vi "uService GUI.vi"(8 "error in (no error)":errorcluster, 11 "uService Test in":refnum<class "test_us.lvclass">) -> (3 "uService Test out":refnum<class "test_us.lvclass">)   [LabVIEW 2026, in "test_us.lvlib" / "test_us.lvclass"]
uses:
  test_us.lvclass
  C:/LabVIEW Code/TALOS/talos/Father of all uServices/Father of all uServices/Father of all uServices.lvclass
  Ancestor/Ancestor/Ancestor.lvclass/Ancestor.ctl
  Support VIs/Substitute Error.vi
  Support VIs/Generate Error.vi
  FGV/Error Memory/Get Error Description.vi
  Support VIs/Get PC name.vi
  Ancestor/Ancestor/Read ID.vi
  Support VIs/Get Class Name.vi
  FGV/Error Memory/Error Memory Core.vi
  <vilib>/AdvancedString/Delimited String to 1D String Array.vi
  <vilib>/AdvancedString/Delimited String to 1D String Array (string).vi
  Support VIs/Circus Root Path.vi
  FGV/Error Memory/Error Crt Lvl checker.vi
  FGV/Error Memory/Error Memory Core.vi/40c8088d-b597-4017-91af-faa98e00292e.vi
  FGV/Error Memory/Error Memory Core.vi/d4a3ab98-063c-4e44-b43d-fbdcfe6c2be2.vi
  Father of all uServices/Father of all uServices/Father of all uServices.lvclass
  C:/LabVIEW Code/TALOS/builds/Actor Framework PPL/Actor Framework.lvlibp/1abvi3w/vi.lib/ActorFramework/Actor/Actor.lvclass
  builds/Actor Framework PPL/Actor Framework.lvlibp/1abvi3w/vi.lib/ActorFramework/Actor/Read Self Enqueuer.vi
  builds/Actor Framework PPL/Actor Framework.lvlibp/1abvi3w/vi.lib/ActorFramework/Stop Msg/Send Normal Stop.vi
  Support VIs/Global Memory.vi
  <vilib>/Utility/LVClass/Get LV Class Name.vi
  Support VIs/Is in Packed Library.vi
  Support VIs/TALOS Root path.vi
  Support VIs/Read CSV worksheet.vi
  Support VIs/Global Constants.vi
  <vilib>/Utility/error.llb/General Error Handler.vi
  Support VIs/Error Log.vi
  Ancestor/Ancestor/Ancestor.lvclass
  <vilib>/Comparison/Equal/Equal Functor/Equal Functor.lvclass
panel:
  in  "stop New uService":bool
  in  "Tab Control":T1(tab)
  in  "Send I exist":bool
  in  "Stop Pat":bool
  in  "Set Guardian Dead":bool
  in  "Snooze VI":bool
  in  "Switch uS View":bool
  out "Message Received":string
  in  "Message to myself":string
  in  "Send":bool
  in  "SEND to Guardian":bool
  in  "Delayed message":bool
  in  "Delay [s]":dbl
  out "Delay submit time":timestamp format="%<%x %.3X>T"
  out "Delay executed":timestamp format="%<%x %.3X>T"
  out "Test Infinite Message":u32
  in  "Start Infinite":bool
  in  "Check Infinite":bool
  in  "Stop Infinite":bool
  out "Infinite?":bool
  in  "send error":bool
  in  "error":errorcluster
  in  "Error code to filter":i32
  in  "Repetitions":i32
  in  "Time (s)":dbl
  in  "Filter error":bool
  in  "Update Run Number":bool
  in  "Run Number":u32
  in  "Send to DAQ":bool
  in  "Add point":bool
  out "LED":bool
  out "Waveform Chart":waveform(dbl)(graph)
  in  "Reset Graph":bool
  out "Counter":dbl
  in  "Set N":bool
  in  "N":i32
  in  "Read N":bool
  out "N out":i32
  out "Safe Mode":bool
  out "uService ID":string
  # "I'm the test uService!"
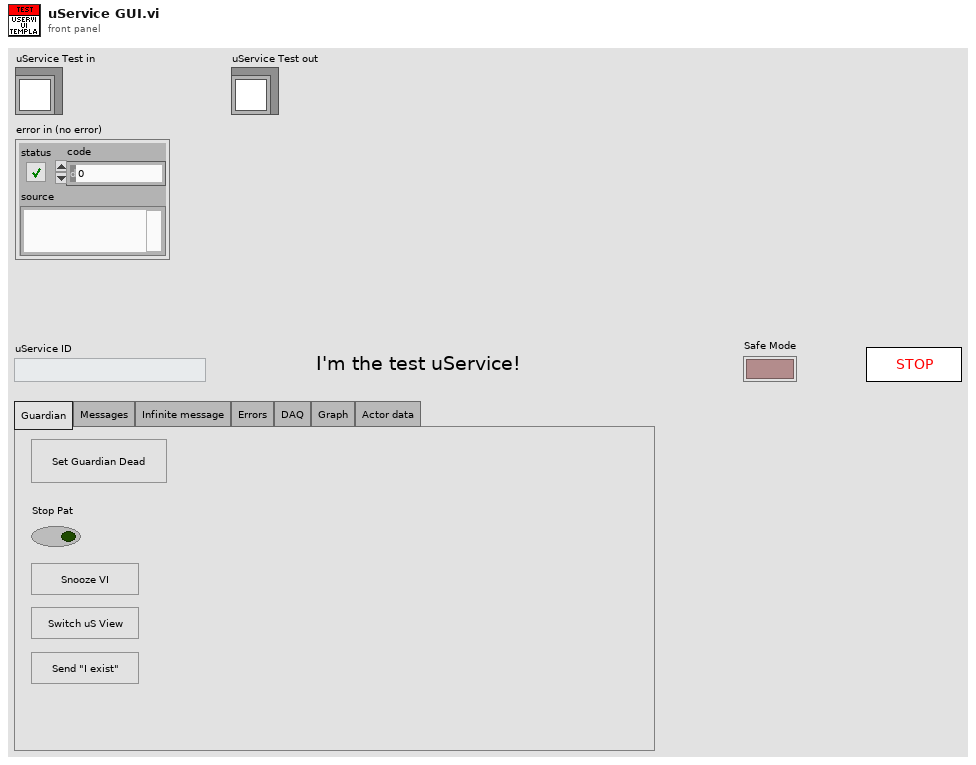
[diagram p1: front panel]
types:
  T1 = enum32{"Guardian", "Messages", "Infinite message", "Errors", "DAQ", "Graph", "Actor data"}
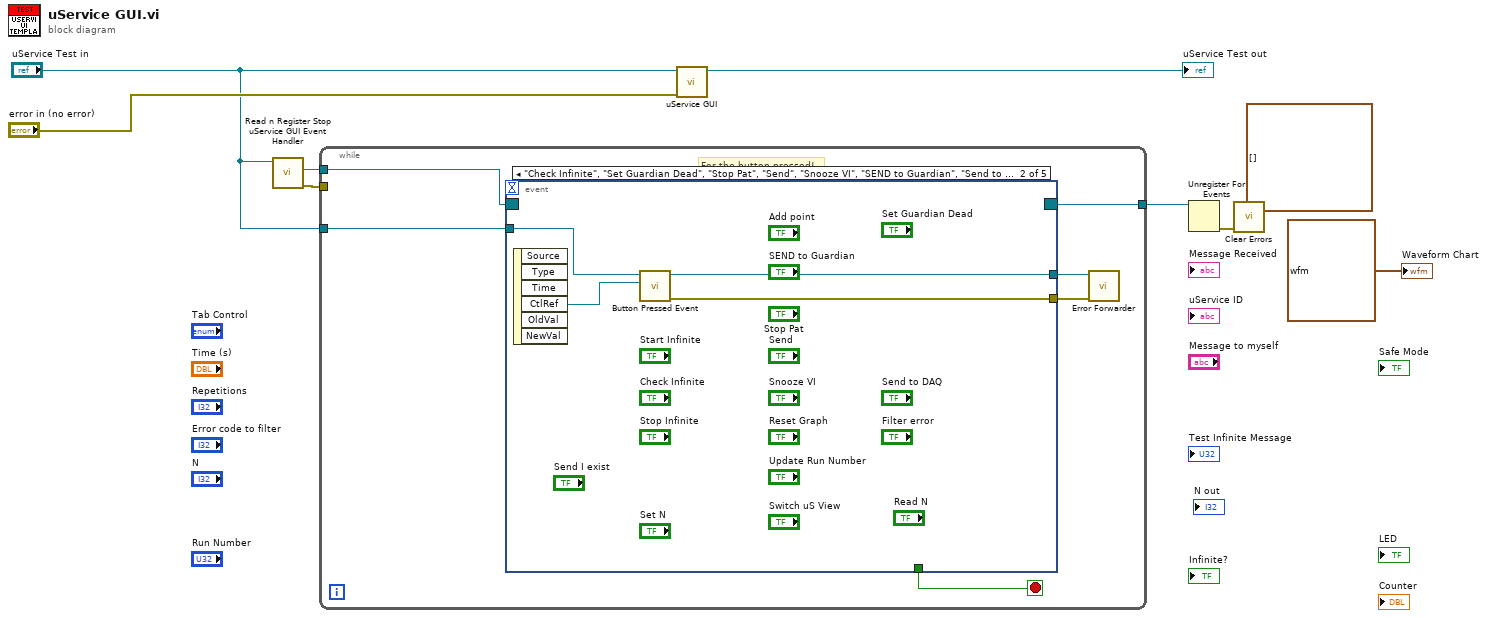
[diagram p0: block diagram]
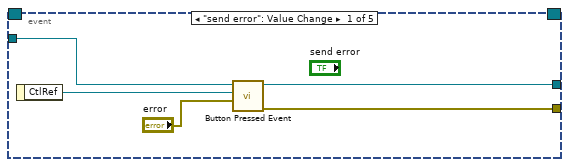
[diagram p2: hidden frame]
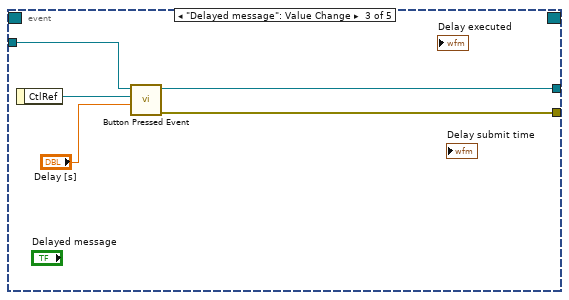
[diagram p3: hidden frame]
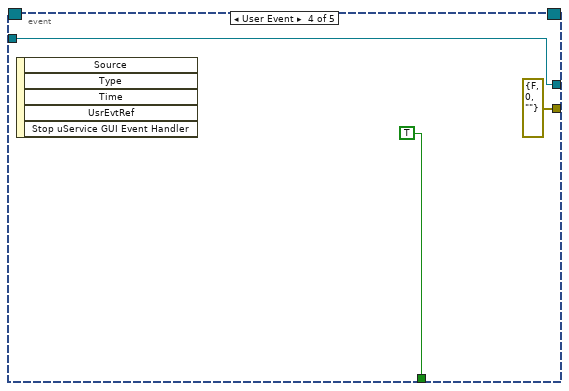
[diagram p4: hidden frame]
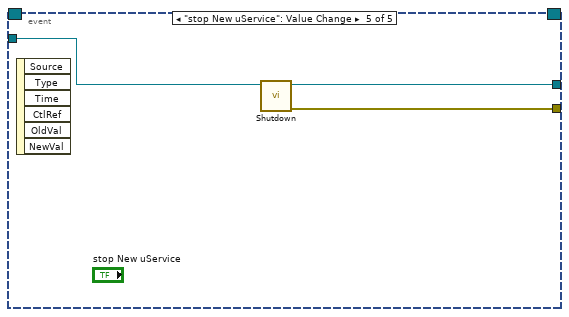
[diagram p5: hidden frame]
diagram:
  (unwired) waveform(dbl)[] []
  n1 = call-dynamic "Read n Register Stop uService GUI Event Handler .vi"("uService Template in"="uService Test in") -> ("error out"=w5:errorcluster, "Stop uService GUI Event Ref"=w4:refnum<event-registration>)  [unwired: 8 in, 1 out]
  n2 = while {
    tunnel: [w14] -> w7
    tunnel: w5 -> [_]
    tunnel: "uService Test in" -> [w12]
    tunnel: w4 -> [w11]
    stop <- w13 stop-if-true
    # "For the button pressed!"
    n3 = event shown="[1] \"Check Infinite\", \"Set Guardian Dead\", \"Stop Pat\", \"Send\", \"Snooze VI\", \"SEND to Guardian\", \"Send to DAQ\", \"Add point\", \"Reset Graph\", \"Start Infinite\", \"Stop Infinite\", \"Filter error\", \"Update Run Number\", \"Set N\", \"Read N\", \"Switch uS View\", \"Send I exist\": Value Change" {
      selector: w11 -> [_ _ _ _ _]
      dyn-events: [_ _ _ _ _] -> w14
      timeout: _ -> [_ _ _ _ _]
      tunnel: w12 -> [w19 w23 w27 w30 w34]
      tunnel: [_ _ _ TRUE _] -> w13
      tunnel: [w16 w21 w25 w30 w33] -> w10
      tunnel: [w15 w20 w24 errorcluster {"status"=FALSE, "code"=0, "source"=""} ("error out") w32] -> w9
      event "send error": Value Change {
        n4 = event-data() -> ("CtlRef"=w18:refnum<vi>)  [unwired: 1 in]
        n5 = call-dynamic "Button Pressed Event.vi"("Data"="error", "CtlRef"=w18, "uService Template in"=w19) -> ("error out"=w15:errorcluster, "uService Template out"=w16:refnum<class "test_us.lvclass">)  [unwired: 7 in]
      }
      event "Check Infinite", "Set Guardian Dead", "Stop Pat", "Send", "Snooze VI", "SEND to Guardian", "Send to DAQ", "Add point", "Reset Graph", "Start Infinite", "Stop Infinite", "Filter error", "Update Run Number", "Set N", "Read N", "Switch uS View", "Send I exist": Value Change {
        n6 = event-data() -> ("CtlRef"=w22:refnum<vi>)  [unwired: 1 in, 5 out]
        n7 = call-dynamic "Button Pressed Event.vi"("CtlRef"=w22, "uService Template in"=w23) -> ("error out"=w20:errorcluster, "uService Template out"=w21:refnum<class "test_us.lvclass">)  [unwired: 8 in]
      }
      event "Delayed message": Value Change {
        n8 = event-data() -> ("CtlRef"=w28:refnum<vi>)  [unwired: 1 in]
        n9 = call-dynamic "Button Pressed Event.vi"("Data"="Delay [s]", "CtlRef"=w28, "uService Template in"=w27) -> ("error out"=w24:errorcluster, "uService Template out"=w25:refnum<class "test_us.lvclass">)  [unwired: 7 in]
      }
      event User Event {
        n10 = event-data() -> ()  [unwired: 1 in, 5 out]
      }
      event "stop New uService": Value Change {
        n11 = event-data() -> ()  [unwired: 1 in, 6 out]
        n12 = call "Shutdown.vi"("Father of all uServices in"=w34) -> ("error out"=w32:errorcluster, "Father of all uServices out"=w33:refnum<class "test_us.lvclass">)  [unwired: 9 in]
      }
    }
    n13 = call "Error Forwarder.vi"("error in (no error)"=w9, "Father of all uServices in"=w10) -> ()  [unwired: 10 in]
  }
  n14 = call-parent "uService GUI.vi"("error in (no error)"="error in (no error)", "uService Template in"="uService Test in") -> ("uService Template out"=→"uService Test out":refnum<class "test_us.lvclass">)  [unwired: 9 in]
  n15 = Unregister For Events(event registration refnum=w7) -> (error out=w2:errorcluster)  [unwired: 1 in]
  n16 = call <vilib>:"Clear Errors.vi"("error in (no error)"=w2) -> ()  [unwired: 5 in, 2 out]
  "Waveform Chart" <- waveform(dbl) {"t0"=timestamp(0 s since 1904-01-01), "dt"=1.0, "Y"=[]} ("Waveform Chart")
